vi "3.2.vi"() -> ()   [LabVIEW 2017]
panel:
  out "result":dbl
  in  "B":dbl
  in  "A":dbl
  in  "功能选择":enum16{"相乘", "相除", "相减", "相加"}(ring)
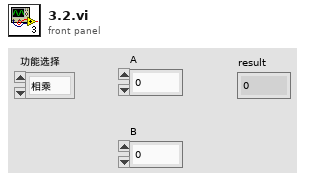
[diagram p1: front panel]
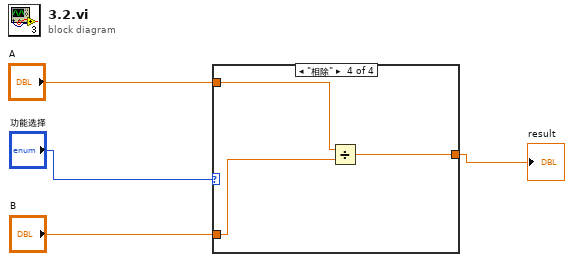
[diagram p0: block diagram]
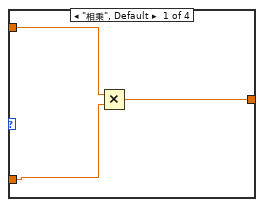
[diagram p2: hidden frame]
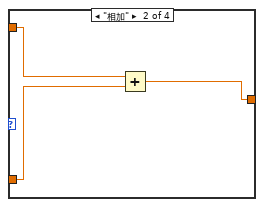
[diagram p3: hidden frame]
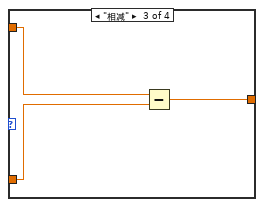
[diagram p4: hidden frame]
diagram:
  n1 = case shown="\"相除\"" "功能选择" {
    tunnel: "B" -> [w5 w8 w11 w15]
    tunnel: [w7 w10 w13 w16] -> w1
    tunnel: "A" -> [w6 w9 w12 w14]
    frame "相乘", Default {
      n2 = Multiply(x=w6, y=w5) -> (x*y=w7:dbl)
    }
    frame "相加" {
      n3 = Add(x=w9, y=w8) -> (x+y=w10:dbl)
    }
    frame "相减" {
      n4 = Subtract(x=w12, y=w11) -> (x-y=w13:dbl)
    }
    frame "相除" {
      n5 = Divide(x=w14, y=w15) -> (x/y=w16:dbl)
    }
  }
  "result" <- w1
